vi "SL TAGS Open Tag.vi"(8 "error in (no error)":errorcluster, 10 "Tag Properties":T1={"Class Data Type"=enum."Double", "Name"="", "Description"="", "Interpolation Method"=enum."linear", "Unit of Measure"=enum."Hour", "Maximum Interpolation"="", "Role"=enum."Supervisor"}, 11 "EEISysLink in":refnum<class "EEISysLink.lvclass">) -> (0 "error out":errorcluster, 3 "EEISysLink out":refnum<class "EEISysLink.lvclass">)   [LabVIEW 2017, in "EEISysLink.lvclass"]
doc: "Will input tag properties and open a local tag object instance. If success it will add to the tag list in the class data. \n\nJames Tillett P.E.\nEndeavor Engineering\nwww.endeavoreng.com"
uses:
  EEISysLink.lvclass
  Controls/SL Tag Properties.ctl
  Controls/SL Tag Data Type.ctl
  Controls/SL Tag Interpolation Method.ctl
  Controls/SL Tag Unit of Measure.ctl
  Controls/SL Tag Type.ctl
  Controls/SL Tag.ctl
  <vilib>/Skyline/Tag/Wrapper/Wrapper_class/NI Skyline Tag.lvclass
  <vilib>/Skyline/Tag/Shared/typedefs/Tag Cluster.ctl
  <vilib>/Skyline/Tag/Shared/typedefs/DataType.ctl
  <vilib>/Skyline/Configuration/Configuration AMQP_class/NI Skyline Configuration AMQP.lvclass
  EEISysLink.lvclass/EEISysLink.ctl
  <vilib>/Skyline/Tag/Wrapper/Wrapper AMQP_class/Open Tag AMQP.vi
  <vilib>/Skyline/Tag/Shared/NI Skyline Tag.lvlib
  <vilib>/Skyline/Tag/Wrapper/Wrapper AMQP_class/NI Skyline Tag AMQP.lvclass
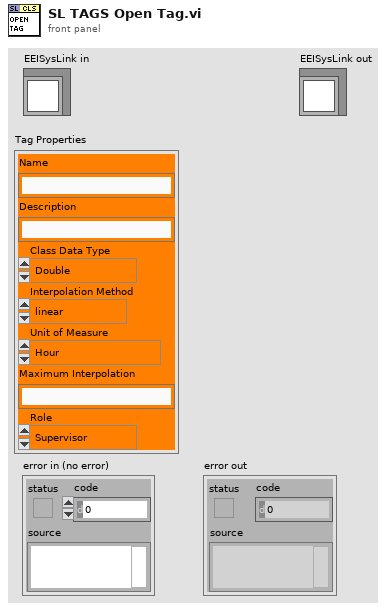
[diagram p1: front panel]
types:
  T1 = typedef "EEISysLink.lvclass/SL Tag Properties.ctl" = cluster{"Class Data Type":T2, "Name":string, "Description":string, "Interpolation Method":T3, "Unit of Measure":T4, "Maximum Interpolation":string, "Role":T5}
  T2 = typedef "EEISysLink.lvclass/SL Tag Data Type.ctl" = enum16{"Double", "Integer", "String", "Boolean", "Waveform"}
  T3 = typedef "EEISysLink.lvclass/SL Tag Interpolation Method.ctl" = enum16{"linear", "pilinear", "step"}
  T4 = typedef "EEISysLink.lvclass/SL Tag Unit of Measure.ctl" = enum16{"no units", "Second", "Hour", "Minute", "Day", "Year", "Month", "Week", "Foot", "Yard", "Meter", "Centimeter", "Inch", "Mile", "Nautical Mile", "Miles per Hour", "Meters per second", "Square meter", "Cubic meter", "Cubic centimeter", "Cubic inch", "Liter", "Gallon", "Gallons dry US", "Gallon UK", "Percent", "Revolutions per minute", "Revolution", "Degree angle", "Astronomical Unit", "Atom", "Atomic mass", "Bar", "Byte", "C (speed of light)", "Curie", "Decibel", "Electron Volt", "Ounce", "Knot", "G", "Grade", "Are", "Hectare", "Faraday", "Franklin", "Gilbert", "Erg", "Lambert", "Maxwell", "Gauss", "Electron mass", "Kilogram force", "Pound force", "Rad", "Centiradian", "Sphere", "Mach", "Fluid Ounces", "Fluid Ounces UK", "Fahrenheit", "Celsius", "Kelvin", "Rankine", "Gram", "Kilogram", "Pound", "Short/US Ton", "Long/UK ton", "Metric ton", "Mole", "Pounds per square inch", "Inches water column", "Torr", "Millitorr", "Millimeter mercury", "Inches mercury", "Bar (2)", "Atmosphere", "Pascal", "Watt", "kiloWatt", "Horsepower", "Kilowatt Hour", "British thermal units", "Millions of BTU", "Ampere", "Candela", "Radian", "Steradian", "Bit", "Hertz", "Newton", "Joule", "Coulomb", "Volt", "Farad", "Ohm", "Siemens", "Weber", "Tesla", "Henry", "Lumen", "Lux", "Becqueral", "Gray", "Sievert", "Katal", "Angstrom", "Light Year", "Parsec", "Point", "Pixel", "Dyne", "Kilogram force (2)", "Pound force (2)", "Rem", "Rutherford", "Roentgen"}
  T5 = typedef "EEISysLink.lvclass/SL Tag Type.ctl" = enum16{"All", "Supervisor", "Worker"}
  T6 = typedef "EEISysLink.lvclass/SL Tag.ctl" = cluster{"Class Properties":T1, "SL Tag":refnum<class "NI Skyline Tag.lvclass">, "SystemLink Cluster":T7, "Class Value":variant}
  T7 = typedef "NI Skyline Tag.lvlib/Tag Cluster.ctl" = cluster{"Path":string, "Data Type":T8, "Value":variant, "Time Stamp":timestamp}
  T8 = typedef "NI Skyline Tag.lvlib/DataType.ctl" = enum32{"Double", "Integer", "String"}
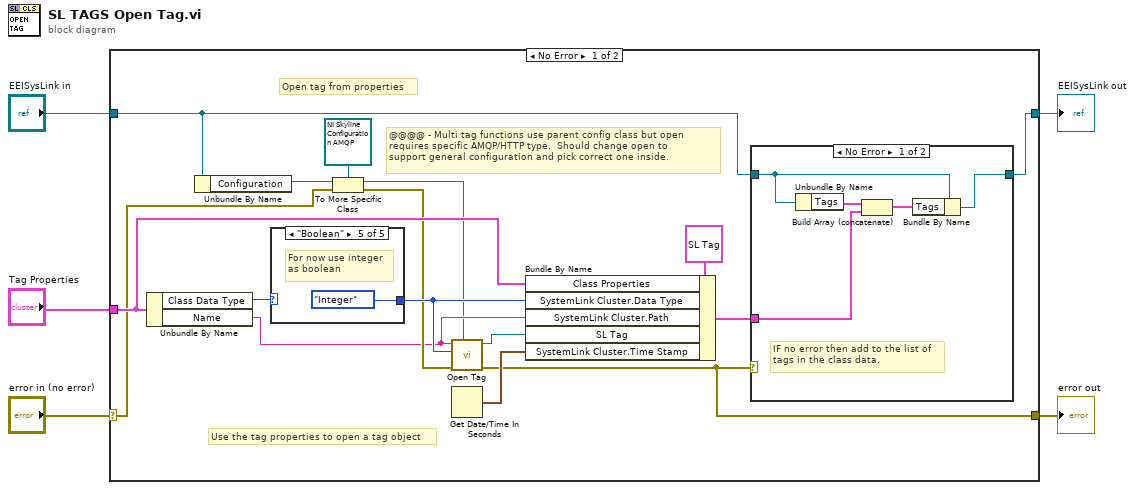
[diagram p0: block diagram]
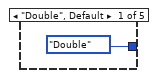
[diagram p3: hidden frame]
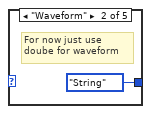
[diagram p4: hidden frame]
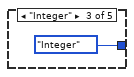
[diagram p5: hidden frame]
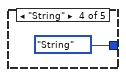
[diagram p6: hidden frame]
diagram:
  n1 = case shown="No Error" "error in (no error)" {
    selector: "error in (no error)" -> [w9 w34]
    tunnel: [w12 w34] -> w4
    tunnel: [w17 w33] -> w2
    tunnel: "EEISysLink in" -> [w15 w33]
    tunnel: "Tag Properties" -> [w16 _]
    frame No Error {
      # "@@@@ - Multi tag functions use parent config class but open\nrequires specific AMQP/HTTP type.  Should change open to\nsupport general configuration and pick correct one inside."
      # "Use the tag properties to open a tag object"
      # "Open tag from properties"
      n2 = Unbundle By Name(w16) -> ("Class Data Type"=w20:T2, "Name"=w7:string)
      n3 = Unbundle By Name(w15) -> ("Configuration"=w11:refnum<class "NI Skyline Configuration.lvclass">)
      n4 = case shown="\"Boolean\"" w20 {
        tunnel: [DataType."Double" ("data type") DataType."String" ("data type") DataType."Integer" ("data type") DataType."String" ("data type") DataType."Integer" ("data type")] -> w14
        frame "Double", Default {
        }
        frame "Waveform" {
          # "For now just use\ndoube for waveform"
        }
        frame "Integer" {
        }
        frame "String" {
        }
        frame "Boolean" {
          # "For now use integer\nas boolean"
        }
      }
      n5 = To More Specific Class(target class=refnum<class "NI Skyline Configuration AMQP.lvclass"> refnum ("configuration"), reference=w11, error in=w9) -> (specific class reference=w6:refnum<class "NI Skyline Configuration AMQP.lvclass">, error out=w8:errorcluster)
      n6 = call-poly <vilib>:"Open Tag.vi"("configuration"=w6, "error in (no error)"=w8, "data type"=w14, "path"=w7) -> ("error out"=w12:errorcluster, "tag out"=w13:refnum<class "NI Skyline Tag.lvclass">)  [unwired: 6 in]
      n7 = Get Date/Time In Seconds() -> (seconds since 1Jan1904=w21:timestamp)
      n8 = Bundle By Name(cluster=T6 {"Class Properties"={"Class Data Type"=enum."Double", "Name"="", "Description"="", "Interpolation Method"=enum."linear", "Unit of Measure"=enum."Hour", "Maximum Interpolation"="", "Role"=enum."Supervisor"}, "SL Tag"=refnum, "SystemLink Cluster"={"Path"="", "Data Type"=enum."Double", "Value"=variant, "Time Stamp"=timestamp(0 s since 1904-01-01)}, "Class Value"=variant} ("Tag"), "Class Properties"=w16, "SystemLink Cluster.Data Type"=w14, "SystemLink Cluster.Path"=w7, "SL Tag"=w13, "SystemLink Cluster.Time Stamp"=w21) -> (w19:T6)
      n9 = case shown="No Error" w12 {
        tunnel: w15 -> [w24 w27]
        tunnel: w19 -> [w25 _]
        tunnel: [w22 w27] -> w17
        frame No Error {
          # "IF no error then add to the list of\ntags in the class data."
          n10 = Unbundle By Name(w24) -> ("Tags"=w26:T6[])
          n11 = Build Array (concatenate)(w26, w25) -> (w23:T6[])
          n12 = Bundle By Name(cluster=w24, "Tags"=w23) -> (w22:refnum<class "EEISysLink.lvclass">)
        }
        frame Error {
          # "Error so don't add to the tag list"
        }
      }
    }
    frame Error {
    }
  }
  "error out" <- w4
  "EEISysLink out" <- w2
